vi "Write to File Shift Information ver2.vi"(4 "Shift Hour Data":u32[][](array[numeric]), 6 "Reject":u32, 7 "Shift":string, 8 "error in":errorcluster, 9 "Actual Per Shift":u32, 10 "FTT Reject":u32, 11 "Refnum in":T1) -> (0 "error out":errorcluster, 3 "refnum out":T1)   [LabVIEW 2018]
uses:
  <vilib>/Utility/config.llb/Config Data RefNum.ctl
  <vilib>/Utility/config.llb/Write Key (U32).vi
  <vilib>/Utility/config.llb/Write Key (String).vi
  <vilib>/Utility/config.llb/NI_LVConfig.lvlib
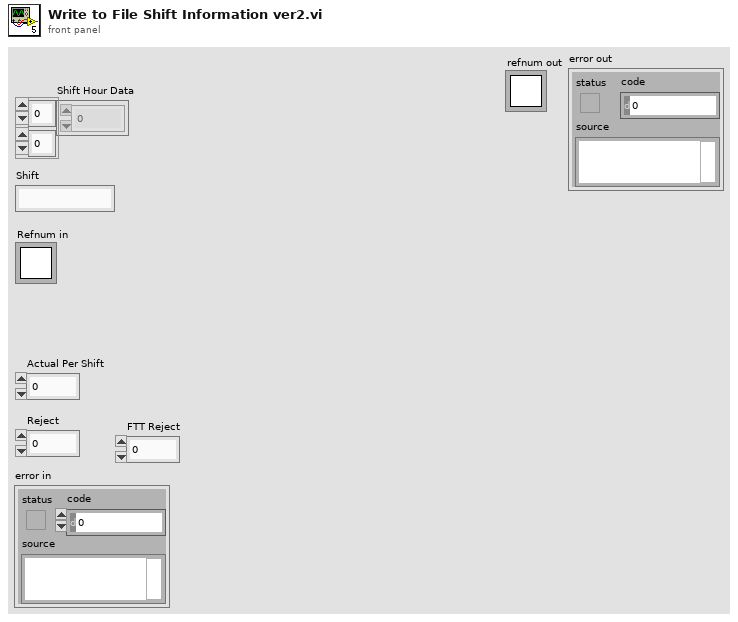
[diagram p1: front panel]
types:
  T1 = typedef "NI_LVConfig.lvlib/Config Data RefNum.ctl" = refnum<k1>
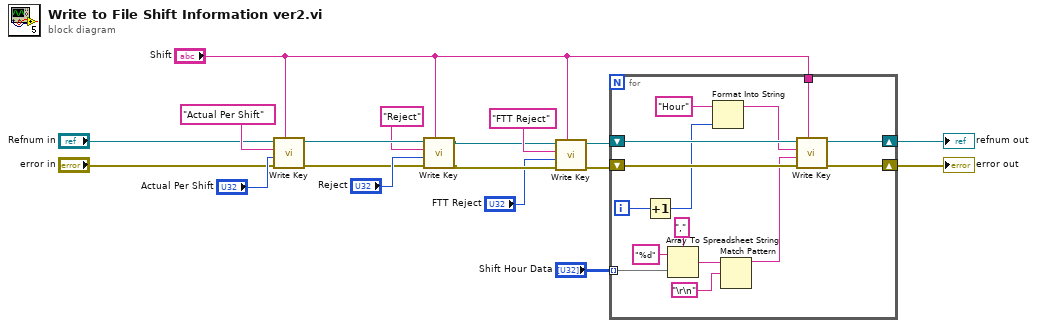
[diagram p0: block diagram]
diagram:
  n1 = call-poly <vilib>:"Write Key.vi"("section"="Shift", "error in (no error)"="error in", "value"="Actual Per Shift", "key"="Actual Per Shift", "refnum"="Refnum in") -> ("error out"=w16:errorcluster, "refnum out"=w15:T1)  [unwired: 4 in, 1 out]
  n2 = call-poly <vilib>:"Write Key.vi"("section"="Shift", "error in (no error)"=w16, "value"="Reject", "key"="Reject", "refnum"=w15) -> ("error out"=w6:errorcluster, "refnum out"=w5:T1)  [unwired: 4 in, 1 out]
  n3 = call-poly <vilib>:"Write Key.vi"("section"="Shift", "error in (no error)"=w6, "value"="FTT Reject", "key"="FTT Reject", "refnum"=w5) -> ("error out"=w3:errorcluster, "refnum out"=w4:T1)  [unwired: 4 in, 1 out]
  n4 = for {
    shift-right: [w27] -> w11
    shift-left: w4 -> [w33]
    shift-right: [w26] -> w10
    shift-left: w3 -> [w32]
    tunnel: "Shift" -> [w31]
    tunnel: "Shift Hour Data" -> [w22] mode=indexing
    i -> [w28]
    n5 = Increment(x=w28) -> (x+1=w25:i32)
    n6 = Array To Spreadsheet String(delimiter (Tab)=",", array=w22, 3:"%d" ("format string")) -> (spreadsheet string=w20:string)
    n7 = Format Into String(initial string="Hour" ("key"), w25) -> (resulting string=w29:string)  [unwired: 2 in, 1 out]
    n8 = Match Pattern(string=w20, regular expression="\r\n") -> (before substring=w19:string)  [unwired: 1 in, 3 out]
    n9 = call-poly <vilib>:"Write Key.vi"("section"=w31, "error in (no error)"=w32, "value"=w19, "key"=w29, "refnum"=w33) -> ("error out"=w26:errorcluster, "refnum out"=w27:T1)  [unwired: 4 in, 1 out]
  }
  "refnum out" <- w11
  "error out" <- w10
